vi "Open System.vi"(4 "Clear Previous Connections (False)":bool, 6 "ID Query (True)":bool, 7 "IP Address":string, 8 "error in (no error)":errorcluster, 9 "Serial Configuration":T4={"Baud Rate"=9600, "Parity"=0, "Data Bits"=8, "Stop Bits"=10, "Flow Control"=0} {"Flow Control" items=["None", "XON/XOFF", "RTS/CTS", "XON/XOFF & RTS/CTS", "DTR/DSR", "XON/XOFF & DTR/DSR"]; "Stop Bits" items=["1.0"=10, "2.0"=20]; "Data Bits" items=["7"=7, "8"=8]; "Parity" items=["None", "Odd", "Even"]; "Baud Rate" items=["300"=300, "600"=600, "1200"=1200, "2400"=2400, "4800"=4800, "9600"=9600, "19200"=19200]}, 10 "Comms Layer":T2, 11 "VISA resource name":refnum<visa-resource-name>) -> (0 "error out":errorcluster, 1 "# of Instruments":i32, 2 "Serial Number(s)":string[](array[string]), 3 "Mercury Reference Out":T1, 5 "S/W Version(s)":string[](array[string]))   [LabVIEW 2019, in "Mercury iXX.lvlib" / "System.lvlib"]
doc: "Opens communication with a Mercury instrument on the chosen communication bus."
uses:
  System.lvlib
  Controls/Serial Settings.ctl
  Controls/Comms Transport Layer.ctl
  Controls/Mercury Reference.ctl
  Private/Controls/Query Dynamic Reference.ctl
  Private/Controls/Lookup Reference FGV Enum.ctl
  <vilib>/Instr/_visa.llb/VISA Flush IO Buffer Mask.ctl
  Mercury iXX.lvlib
panel:
  in  "Reset (True)":bool
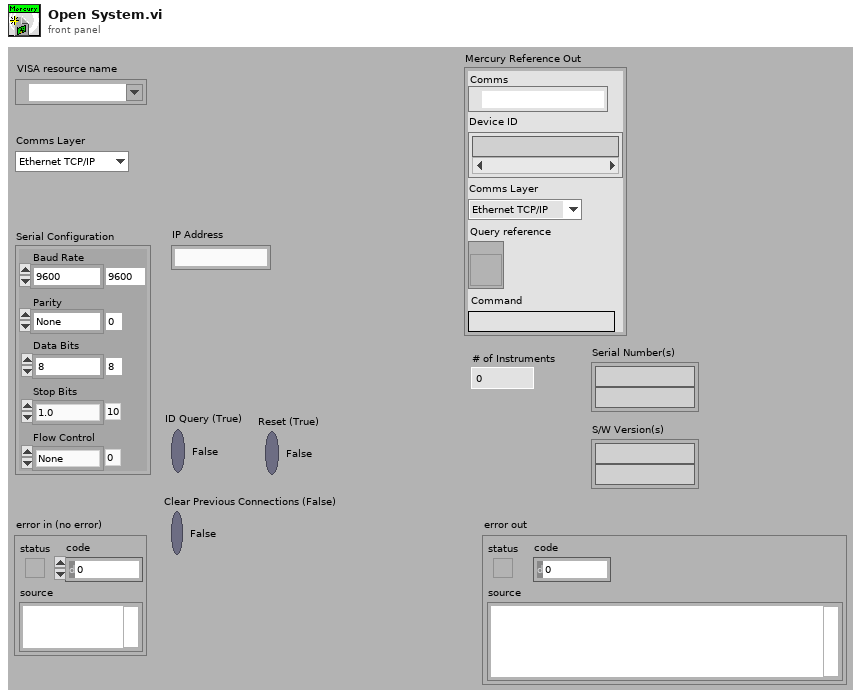
[diagram p1: front panel]
types:
  T1 = typedef "Mercury iXX.lvlib/Mercury Reference.ctl" = cluster{"Comms":refnum<visa-resource-name>, "Device ID":string[], "Comms Layer":T2, "Command":string, "Query reference":T3}
  T2 = typedef "Mercury iXX.lvlib/Comms Transport Layer.ctl" = enum16{"Ethernet TCP/IP", "USB", "ISOBus - RS-232", "GPIB"}
  T3 = typedef "Mercury iXX.lvlib/Query Dynamic Reference.ctl" = refnum<vi>
  T4 = typedef "Mercury iXX.lvlib/Serial Settings.ctl" = cluster{"Baud Rate":u32, "Parity":u16, "Data Bits":u16, "Stop Bits":u16, "Flow Control":u16}
  T5 = typedef "Mercury iXX.lvlib/Lookup Reference FGV Enum.ctl" = enum16{"Check VISA", "Get VI Ref", "Set VI ref", "Delete Single Ref", "Clear All"}
  T6 = typedef "VISA Flush IO Buffer Mask.ctl" = u16
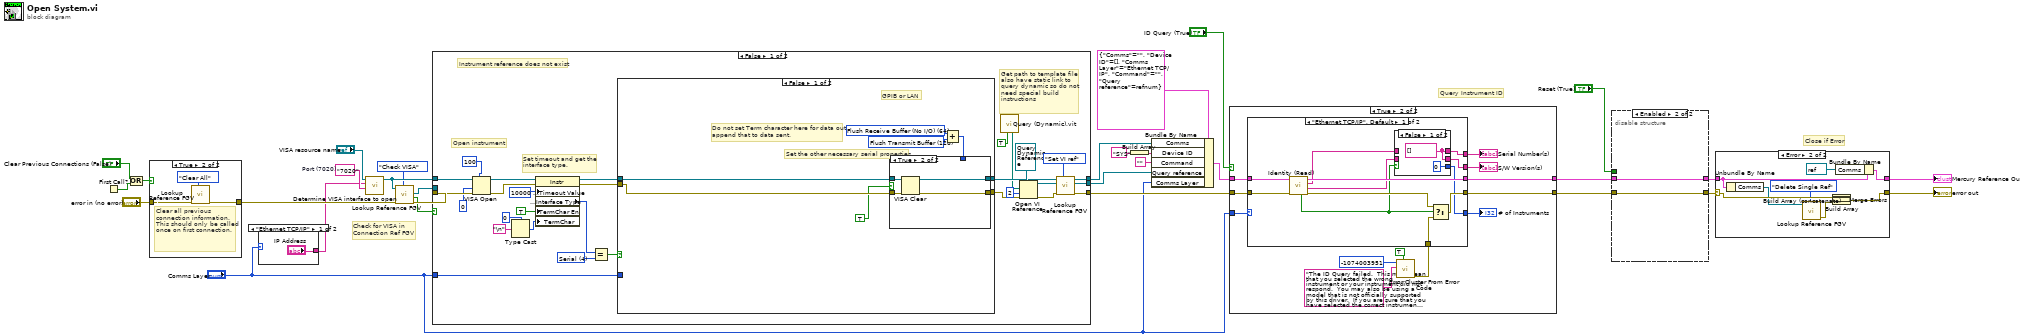
[diagram p0: block diagram]
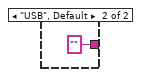
[diagram p2: hidden frame]
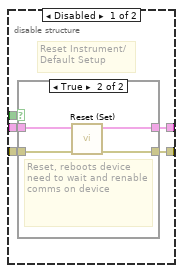
[diagram p4: hidden frame]
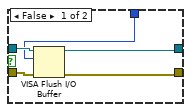
[diagram p6: hidden frame]
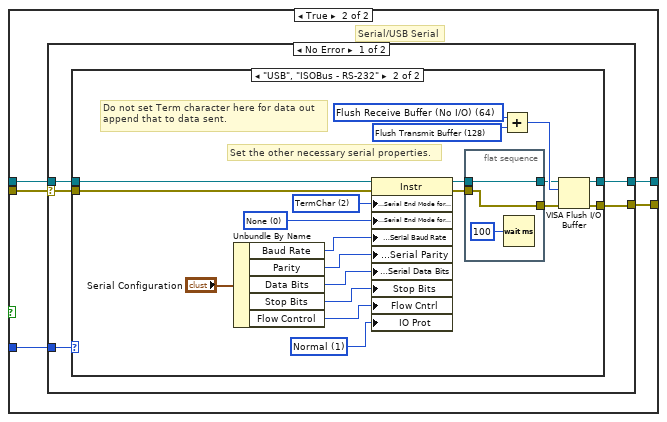
[diagram p7: hidden frame]
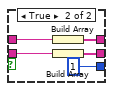
[diagram p13: hidden frame]
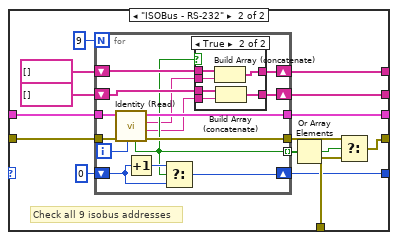
[diagram p14: hidden frame]
diagram:
  w30 = "7020"  # Port (7020)
  # "Check for VISA in \nConnection Ref FGV"
  # "Close if Error"
  # "Query Instrument ID"
  n1 = First Call?() -> (First Call?: T/F=w3:bool)
  n2 = Or(x="Clear Previous Connections (False)", y=w3) -> (x .or. y?=w4:bool)
  n3 = case shown="True" w4 {
    tunnel: "error in (no error)" -> [w31 w34]
    tunnel: [w31 w33] -> w5
    frame False {
    }
    frame True {
      # "Clear all previous connection information. This should only be called once on first connection."
      n4 = call "Lookup Reference FGV.vi"("State"=Lookup_Reference_FGV_Enum."Clear All", "error in"=w34) -> ("error out"=w33:errorcluster)  [unwired: 3 in, 6 out]
    }
  }
  n5 = case shown="\"Ethernet TCP/IP\"" "Comms Layer" {
    tunnel: ["IP Address" "" ("IP Address")] -> w1
    frame "Ethernet TCP/IP" {
    }
    frame "USB", Default {
    }
  }
  n6 = call "Determine VISA interface to open.vi"("Port (7020)"=w30, "IP Address"=w1, "VISA resource name"="VISA resource name") -> ("VISA resource name out"=w12:refnum<visa-resource-name>)  [unwired: 8 out]
  n7 = call "Lookup Reference FGV.vi"("State"=Lookup_Reference_FGV_Enum."Check VISA", "error in"=w5, "VISA In"=w12) -> ("error out"=w13:errorcluster, "Found Ref?"=w9:bool, "Query ref"=w8:T3)  [unwired: 2 in, 4 out]
  n8 = case shown="False" w9 {
    tunnel: w13 -> [w65 w122]
    tunnel: [w43 w122] -> w28
    tunnel: w12 -> [w56 w121]
    tunnel: [w45 w121] -> w16
    tunnel: "Comms Layer" -> [w51 _]
    tunnel: w8 -> [_ w120]
    tunnel: [w47 w120] -> w10
    frame False {
      w61 = u16 4 items=["GPIB"=1, "VXI"=2, "GPIB-VXI"=3, "Serial"=4, "PXI"=5, "TCPIP"=6, "USB"=7] ("Interface Information:Interface Type")
      # "Get path to template file\nalso have static link to \nquery dynamic so do not\nneed special build\ninstructions"
      # "Instrument reference does not exist"
      # "Set timeout and get the\ninterface type."
      # "Open instrument"
      n9 = VISA Open(timeout (0)=100, access mode=u32 0, error in (no error)=w65, VISA resource name=w56) -> (VISA resource name=w59:refnum<visa-resource-name>, error out=w37:errorcluster)  [unwired: 1 out]
      n10 = Type Cast(type=u8 0 ("Message Based Settings:Termination Character"), x="\n") -> (*(type *) &x=w53:u8)
      n11 = property on="Property Node" class="Instr"(reference=w59, error in=w37, "General Settings:Timeout Value"=u32 10000, "TermChar En"=TRUE ("Message Based Settings:Termination Character Enable"), "TermChar"=w53) -> (reference out=w58:refnum<visa-resource-name>, error out=w57:errorcluster, "Interface Information:Interface Type"=w64:u16)
      n12 = Equal?(x=w64, y=w61) -> (x = y?=w62:bool)
      n13 = case shown="False" w62 {
        tunnel: [w71 w87] -> w46
        tunnel: [w70 w86] -> w49
        tunnel: w58 -> [w72 w85]
        tunnel: w57 -> [w73 w84]
        tunnel: w51 -> [_ w83]
        frame False {
          w67 = T6 128 items=["Flush Receive Buffer"=16, "Write Transmit Buffer to Device"=32, "Flush Receive Buffer (No I/O)"=64, "Flush Transmit Buffer"=128] ("Mask")
          w68 = T6 64 items=["Flush Receive Buffer"=16, "Write Transmit Buffer to Device"=32, "Flush Receive Buffer (No I/O)"=64, "Flush Transmit Buffer"=128] ("Mask")
          # "Do not set Term character here for data out append that to data sent."
          # "Set the other necessary serial properties."
          # "GPIB or LAN"
          n14 = Add(x=w68, y=w67) -> (x+y=w66:T6)
          n15 = case shown="True" TRUE {
            tunnel: w73 -> [w77 w82]
            tunnel: w72 -> [w78 w81]
            tunnel: [w76 w80] -> w71
            tunnel: [w75 w79] -> w70
            tunnel: w66 -> [w74 _]
            frame False {
              n16 = VISA Flush I/O Buffer(VISA resource name=w78, mask (16)=w74, error in (no error)=w77) -> (VISA resource name out=w76:refnum<visa-resource-name>, error out=w75:errorcluster)
            }
            frame True {
              n17 = VISA Clear(VISA resource name=w81, error in (no error)=w82) -> (VISA resource name out=w80:refnum<visa-resource-name>, error out=w79:errorcluster)
            }
          }
        }
        frame True {
          # "Serial/USB Serial"
          n18 = case shown="No Error" w84 {
            tunnel: w85 -> [w90 w119]
            selector: w84 -> [w89 w118]
            tunnel: [w92 w119] -> w87
            tunnel: [w91 w118] -> w86
            tunnel: w83 -> [w88 _]
            frame No Error {
              n19 = case shown="\"USB\", \"ISOBus - RS-232\"" w88 {
                tunnel: [w94 w102] -> w92
                tunnel: [w93 w103] -> w91
                tunnel: w90 -> [w94 w104]
                tunnel: w89 -> [w93 w106]
                frame "Ethernet TCP/IP", Default {
                }
                frame "USB", "ISOBus - RS-232" {
                  w100 = T6 128 items=["Flush Receive Buffer"=16, "Write Transmit Buffer to Device"=32, "Flush Receive Buffer (No I/O)"=64, "Flush Transmit Buffer"=128] ("Mask")
                  w101 = T6 64 items=["Flush Receive Buffer"=16, "Write Transmit Buffer to Device"=32, "Flush Receive Buffer (No I/O)"=64, "Flush Transmit Buffer"=128] ("Mask")
                  w105 = u16 2 items=["None", "LastBit", "TermChar"] ("Serial Settings:Serial End Mode for Reads")
                  w114 = u16 1 items=["Normal"=1, "VXI/FDC"=2, "GPIB/HS488"=3, "Serial-TCPIP-USB/488 Strings"=4, "USBTMC/Vendor-Specific"=5] ("Message Based Settings:IO Protocol")
                  w109 = u16 0 items=["None", "LastBit", "TermChar"] ("Serial Settings:Serial End Mode for Reads")
                  # "Do not set Term character here for data out append that to data sent."
                  # "Set the other necessary serial properties."
                  n20 = Unbundle By Name("Serial Configuration") -> ("Baud Rate"=w111:u32, "Parity"=w113:u16, "Data Bits"=w112:u16, "Stop Bits"=w108:u16, "Flow Control"=w107:u16)
                  n21 = property on="Property Node" class="Instr"(reference=w104, error in=w106, "Serial Settings:Serial End Mode for Reads"=w105, "Serial Settings:Serial End Mode for Writes"=w109, "Serial Settings:Serial Baud Rate"=w111, "Serial Settings:Serial Parity"=w113, "Serial Settings:Serial Data Bits"=w112, "Stop Bits"=w108, "Flow Cntrl"=w107, "IO Prot"=w114) -> (reference out=w98:refnum<visa-resource-name>, error out=w96:errorcluster)
                  n22 = flat-sequence {
                    tunnel: w98 -> [w116]
                    tunnel: [w116] -> w97
                    tunnel: w96 -> [w115]
                    tunnel: [w115] -> w95
                    frame #0 {
                      n23 = Wait (ms)(milliseconds to wait=u32 100) -> ()  [unwired: 1 out]
                    }
                  }
                  n24 = Add(x=w101, y=w100) -> (x+y=w99:T6)
                  n25 = VISA Flush I/O Buffer(VISA resource name=w97, mask (16)=w99, error in (no error)=w95) -> (VISA resource name out=w102:refnum<visa-resource-name>, error out=w103:errorcluster)
                }
              }
            }
            frame Error {
              # "If there is an error in, do not attempt to set additional serial parameters."
            }
          }
        }
      }
      n26 = call "Query (Dynamic).vit"("Path Only"=TRUE) -> ("path"=w41:path)  [unwired: 5 in, 5 out]
      n27 = Open VI Reference(type specifier VI Refnum (for type only)=T3 refnum ("Query reference"), vi path=w41, options=2, error in (no error)=w49) -> (vi reference=w48:T3, error out=w44:errorcluster)  [unwired: 1 in, 1 out]
      n28 = call "Lookup Reference FGV.vi"("State"=Lookup_Reference_FGV_Enum."Set VI ref", "error in"=w44, "Query ref in"=w48, "VISA In"=w46) -> ("error out"=w43:errorcluster, "Query ref"=w47:T3, "VISA Out"=w45:refnum<visa-resource-name>)  [unwired: 1 in, 4 out]
    }
    frame True {
      # "Read connection ref from FGV"
      # "Instrument Reference Exists."
    }
  }
  n29 = Build Array("SYS") -> (w18:string[])
  n30 = Bundle By Name(cluster=T1 {"Comms"="", "Device ID"=[], "Comms Layer"=enum."Ethernet TCP/IP", "Command"="", "Query reference"=refnum} ("Mercury Reference"), "Comms"=w16, "Device ID"=w18, "Command"="", "Query reference"=w10, "Comms Layer"="Comms Layer") -> (w15:T1)
  n31 = case shown="True" "ID Query (True)" {
    tunnel: [w123 w136] -> w22
    tunnel: [w124 w133] -> w23
    tunnel: w15 -> [w124 w134]
    tunnel: w28 -> [w123 w135]
    tunnel: "Comms Layer" -> [_ w129]
    frame False {
    }
    frame True {
      n32 = call <vilib>:"Error Cluster From Error Code.vi"("show call chain? (False)"=TRUE, "error message (\"\")"="The ID Query failed.  This may mean that you selected the wrong instrument or your instrument did not respond.  You may also be using a model that is not officially supported by this driver.  If you are sure that you have selected the correct instrument and it is responding, try disabling the ID Query." ("Source (VI Name)"), "error code (0)"=-1074003951 ("Code")) -> ("error out"=w132:errorcluster)  [unwired: 1 in, 5 out]
      n33 = case shown="\"Ethernet TCP/IP\", Default" w129 {
        tunnel: [w148 w165] -> w136
        tunnel: w135 -> [w143 w169]
        tunnel: w134 -> [w146 w170]
        tunnel: [w145 w163] -> w133
        tunnel: w132 -> [w147 w167]
        tunnel: [w138 w158] -> w128
        tunnel: [w139 w157] -> w127
        tunnel: [w140 w156] -> w126
        frame "Ethernet TCP/IP", Default {
          n34 = call "Identity (Read).vi"("error in"=w143, "Mercury Reference In"=w146) -> ("error out"=w144:errorcluster, "S/W Version"=w141:string, "Serial Number"=w142:string, "Mercury Reference Out"=w145:T1, "Instrument Valid?"=w137:bool)  [unwired: 1 in, 4 out]
          n35 = case shown="False" w137 {
            tunnel: w142 -> [_ w155]
            tunnel: w141 -> [_ w154]
            tunnel: [w149 w153] -> w140
            tunnel: [w149 w152] -> w139
            tunnel: [0 1] -> w138
            frame False {
              w149 = string[] []
            }
            frame True {
              n36 = Build Array(w155) -> (w152:string[])
              n37 = Build Array(w154) -> (w153:string[])
            }
          }
          n38 = Select(t=w144, s=w137, f=w147) -> (s? t:f=w148:errorcluster)
        }
        frame "ISOBus - RS-232" {
          # "Check all 9 isobus addresses"
          n39 = for {
            N: 9 -> [_]
            tunnel: w170 -> [w185]
            tunnel: w169 -> [w184]
            tunnel: [w182] -> w166
            tunnel: [w173] -> w168 mode=indexing
            tunnel: [w181] -> w163
            shift-right: [w179] -> w158
            shift-left: 0 -> [w178]
            shift-right: [w174] -> w156
            shift-left: string[] [] -> [w175]
            shift-right: [w176] -> w157
            shift-left: string[] [] -> [w177]
            i -> [w183]
            n40 = call "Identity (Read).vi"("ISOBUS address"=w183, "error in"=w184, "Mercury Reference In"=w185) -> ("error out"=w182:errorcluster, "S/W Version"=w171:string, "Serial Number"=w172:string, "Mercury Reference Out"=w181:T1, "Instrument Valid?"=w173:bool)  [unwired: 4 out]
            n41 = Increment(x=w178) -> (x+1=w180:i32)
            n42 = Select(t=w180, s=w173, f=w178) -> (s? t:f=w179:i32)
            n43 = case shown="True" w173 {
              tunnel: w177 -> [w187 w193]
              tunnel: [w187 w192] -> w176
              tunnel: w175 -> [w186 w191]
              tunnel: [w186 w190] -> w174
              tunnel: w172 -> [_ w189]
              tunnel: w171 -> [_ w188]
              frame False {
              }
              frame True {
                n44 = Build Array (concatenate)(w193, w189) -> (w192:string[])
                n45 = Build Array (concatenate)(w191, w188) -> (w190:string[])
              }
            }
          }
          n46 = Or Array Elements(Boolean array=w168) -> (logical OR=w164:bool)
          n47 = Select(t=w166, s=w164, f=w167) -> (s? t:f=w165:errorcluster)
        }
      }
      "Serial Number(s)" <- w127
      "S/W Version(s)" <- w126
      "# of Instruments" <- w128
    }
  }
  n48 = disable-structure shown="Enabled" {
    disable-tunnel: "Reset (True)" -> [w198 _]
    disable-tunnel: [w197 w206] -> w25
    disable-tunnel: [w196 w205] -> w24
    disable-tunnel: w23 -> [w195 w206]
    disable-tunnel: w22 -> [w194 w205]
    frame Disabled {
      # "Reset Instrument/\nDefault Setup"
      n49 = case shown="True" w198 {
        tunnel: w194 -> [w200 w203]
        tunnel: [w200 w201] -> w196
        tunnel: w195 -> [w199 w204]
        tunnel: [w199 w202] -> w197
        frame False {
        }
        frame True {
          # "Reset, reboots device need to wait and renable comms on device"
          n50 = call "Reset (Set).vi"("error in"=w203, "Mercury Reference In"=w204) -> ("error out"=w201:errorcluster, "Mercury Reference Out"=w202:T1)  [unwired: 6 in, 2 out]
        }
      }
    }
    frame Enabled {
    }
  }
  n51 = case shown="Error" w24 {
    selector: w24 -> [w207 w218]
    tunnel: w25 -> [w208 w213]
    tunnel: [w208 w217] -> w14
    tunnel: [w207 w215] -> w21
    frame No Error {
    }
    frame Error {
      n52 = Unbundle By Name(w213) -> ("Comms"=w212:refnum<visa-resource-name>)
      n53 = call "Lookup Reference FGV.vi"("State"=Lookup_Reference_FGV_Enum."Delete Single Ref", "VISA In"=w212) -> ("error out"=w214:errorcluster)  [unwired: 3 in, 6 out]
      n54 = Build Array(w218, w214) -> (w210:errorcluster[])
      n55 = Build Array (concatenate)(w210) -> (w209:errorcluster[])
      n56 = Merge Errors(w209) -> (w215:errorcluster)
      n57 = Bundle By Name(cluster=w213, "Comms"=refnum<visa-resource-name> refnum ("VISA resource name out")) -> (w217:T1)
    }
  }
  "error out" <- w21
  "Mercury Reference Out" <- w14
